vi "Open File.vi"(8 "error in":errorcluster, 11 "CSV in":refnum<class "CSV.lvclass">) -> (0 "error out":errorcluster, 3 "CSV out":refnum<class "CSV.lvclass">)   [LabVIEW 2019, in "ManejoArchivos.lvlib" / "CSV.lvclass"]
uses:
  CSV.lvclass
  C:/GitClones/PowerElectronics/28 Mayo Prueba Plantilla/Libraries/ManejoArchivos/Class Definitions/File/File.lvclass
  CSV.lvclass/CSV.ctl
  File/File.lvclass/File.ctl
  File/Read File Path.vi
  Write file Ref.vi
  Read file Ref.vi
  File/File.lvclass
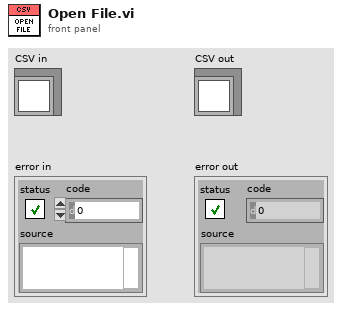
[diagram p1: front panel]
types:
  T1 = enum16{"open", "replace", "create", "open or create", "replace or create", "replace or create with confirmation"}
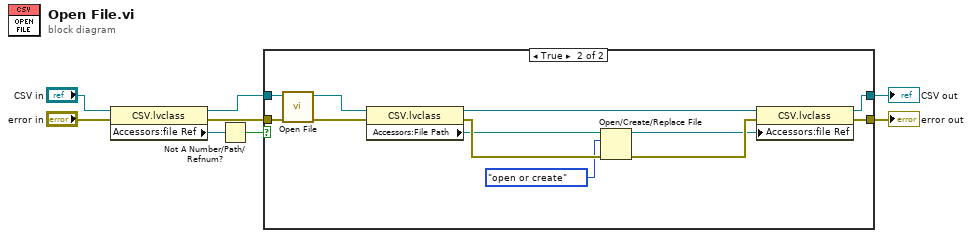
[diagram p0: block diagram]
diagram:
  n1 = property class="CSV.lvclass"(reference="CSV in", error in="error in") -> (reference out=w3:refnum<class "CSV.lvclass">, error out=w5:errorcluster, "Accessors:file Ref"=w2:refnum<file>)
  n2 = Not A Number/Path/Refnum?(number/path/refnum=w2) -> (NaN/Path/Refnum?=w1:bool)
  n3 = case shown="True" w1 {
    tunnel: w5 -> [w10 w22]
    tunnel: [w10 w19] -> w7
    tunnel: w3 -> [w9 w12]
    tunnel: [w9 w14] -> w6
    frame False {
    }
    frame True {
      n4 = call-parent "Open File.vi"("error in"=w22, "File in"=w12) -> ("error out"=w18:errorcluster, "File out"=w11:refnum<class "CSV.lvclass">)  [unwired: 8 in]
      n5 = property class="CSV.lvclass"(reference=w11, error in=w18) -> (reference out=w15:refnum<class "CSV.lvclass">, error out=w21:errorcluster, "Accessors:File Path"=w16:path)
      n6 = Open/Create/Replace File(file path (use dialog)=w16, error in=w21, operation (0:open)=T1."open or create") -> (refnum out=w13:refnum<file>, error out=w20:errorcluster)  [unwired: 3 in, 1 out]
      n7 = property class="CSV.lvclass"(reference=w15, error in=w20, "Accessors:file Ref"=w13) -> (reference out=w14:refnum<class "CSV.lvclass">, error out=w19:errorcluster)
    }
  }
  "error out" <- w7
  "CSV out" <- w6
